vi "Write Header.vi"(10 "Header":string, 11 "CSV File Sink in":refnum<class "CSV File Sink.lvclass">) -> (3 "CSV File Sink out":refnum<class "CSV File Sink.lvclass">)   [LabVIEW 2016, in "Stream Log.lvlib" / "CSV File Sink.lvclass"]
uses:
  <userlib>/Composed Systems/Stream/Log/CSV File Sink/CSV File Sink.lvclass
  <userlib>/Composed Systems/Stream/Log/CSV File Sink/CSV File Sink.lvclass/CSV File Sink.ctl
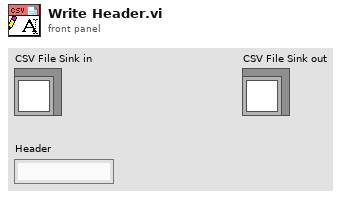
[diagram p1: front panel]
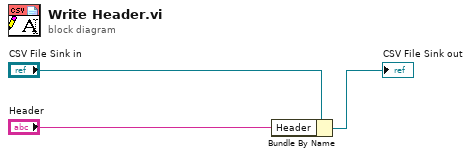
[diagram p0: block diagram]
diagram:
  n1 = Bundle By Name(cluster="CSV File Sink in", "Header"="Header") -> (→"CSV File Sink out":refnum<class "CSV File Sink.lvclass">)
